vi "Get Obstacles.vi"() -> (0 "Obstacles":dbl[](array[numeric]))   [LabVIEW 2015]
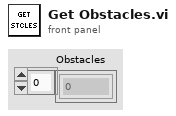
[diagram p1: front panel]
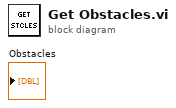
[diagram p0: block diagram]
diagram:
